vi "GetSlideScaleReference.vi"(8 "error in":errorcluster, 11 "SlideScale in":refnum<class "SlideScale.lvclass">) -> (0 "error out":errorcluster, 1 "slide scale reference":refnum<vi>, 3 "SlideScale out":refnum<class "SlideScale.lvclass">)   [LabVIEW 2014, in "Raspberry Pi Compatible Compiler for LabVIEW.lvlib" / "SlideScale.lvclass"]
uses:
  SlideScale.lvclass
  Generic/Generic.lvclass
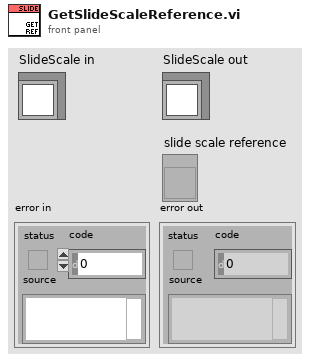
[diagram p1: front panel]
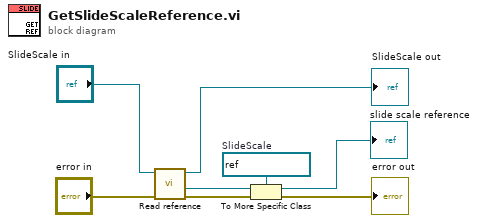
[diagram p0: block diagram]
diagram:
  w5 = refnum<vi> refnum  # SlideScale
  n1 = call "Read reference.vi"("error in"="error in", "GObject in"="SlideScale in") -> ("error out"=w6:errorcluster, "reference"=w7:refnum<vi>, "GObject out"=→"SlideScale out":refnum<class "SlideScale.lvclass">)  [unwired: 5 in]
  n2 = To More Specific Class(target class=w5, reference=w7, error in=w6) -> (specific class reference=→"slide scale reference":refnum<vi>, error out=→"error out":errorcluster)
